vi "TDLAS.vi"() -> ()   [LabVIEW 2016]
uses:
  <vilib>/DAQmx/read.llb/DAQmx Read.vi
  <vilib>/DAQmx/read.llb/DAQmx Read (Analog 1D Wfm NChan NSamp).vi
  <vilib>/DAQmx/create/channels.llb/DAQmx Create Channel (AI-Voltage-Basic).vi
  <vilib>/DAQmx/miscellaneous.llb/DAQmx Fill In Error Info.vi
panel:
  in  "physical channels":tag
  out "data":waveform(dbl)[](graph)
  in  "stop 2":bool caption="stop"
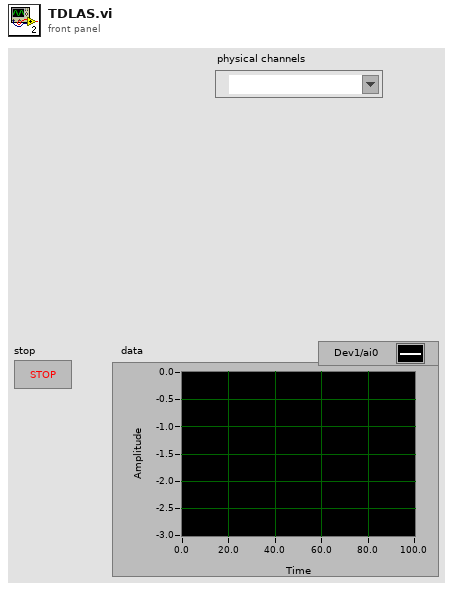
[diagram p1: front panel]
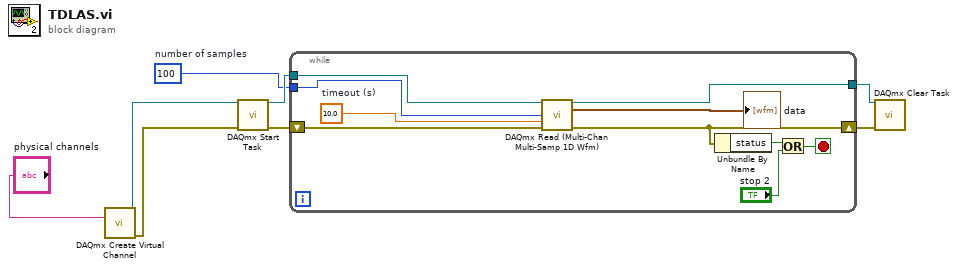
[diagram p0: block diagram]
diagram:
  w6 = 100  # number of samples
  n1 = call-poly <vilib>:"DAQmx Create Virtual Channel.vi"("physical channels"="physical channels") -> ("task out"=w2:refnum<k21>, "error out"=w3:errorcluster)  [unwired: 13 in]
  n2 = call <vilib>:"DAQmx Start Task.vi"("task/channels in"=w2, "error in"=w3) -> ("task out"=w8:refnum<k21>, "error out"=w7:errorcluster)  [unwired: 12 in]
  n3 = while {
    tunnel: w8 -> [w18]
    tunnel: w6 -> [w14]
    tunnel: [w15] -> w4
    shift-right: [w12] -> w5
    shift-left: w7 -> [w17]
    stop <- w11 stop-if-true
    w9 = 10.0  # timeout (s)
    n4 = call-poly "DAQmx Read (Multi-Chan Multi-Samp 1D Wfm).vi"("task/channels in"=w18, "number of samples per channel"=w14, "timeout"=w9, "error in"=w17) -> ("task out"=w15:refnum<k21>, "data"=→"data":waveform(dbl)[], "error out"=w12:errorcluster)  [unwired: 9 in]
    n5 = Unbundle By Name(w12) -> ("status"=w13:bool)
    n6 = Or(x=w13, y="stop 2") -> (x .or. y?=w11:bool)
  }
  n7 = call <vilib>:"DAQmx Clear Task.vi"("task in"=w4, "error in"=w5) -> ()  [unwired: 13 in, 1 out]
